vi "use photons for state.vi"(0 "state in":T1, 1 "apply measurement?":bool, 5 "location":T3, 7 "z-offset":i16, 9 "half valid z-range (ncycles * 64)":i16=500, 11 "scan radius":u16, 12 "tracking":bool) -> (4 "use photons to update tracker?":bool)   [LabVIEW 2010]
uses:
  kalman 3-axis state.ctl
  integrating single axis kalman state.ctl
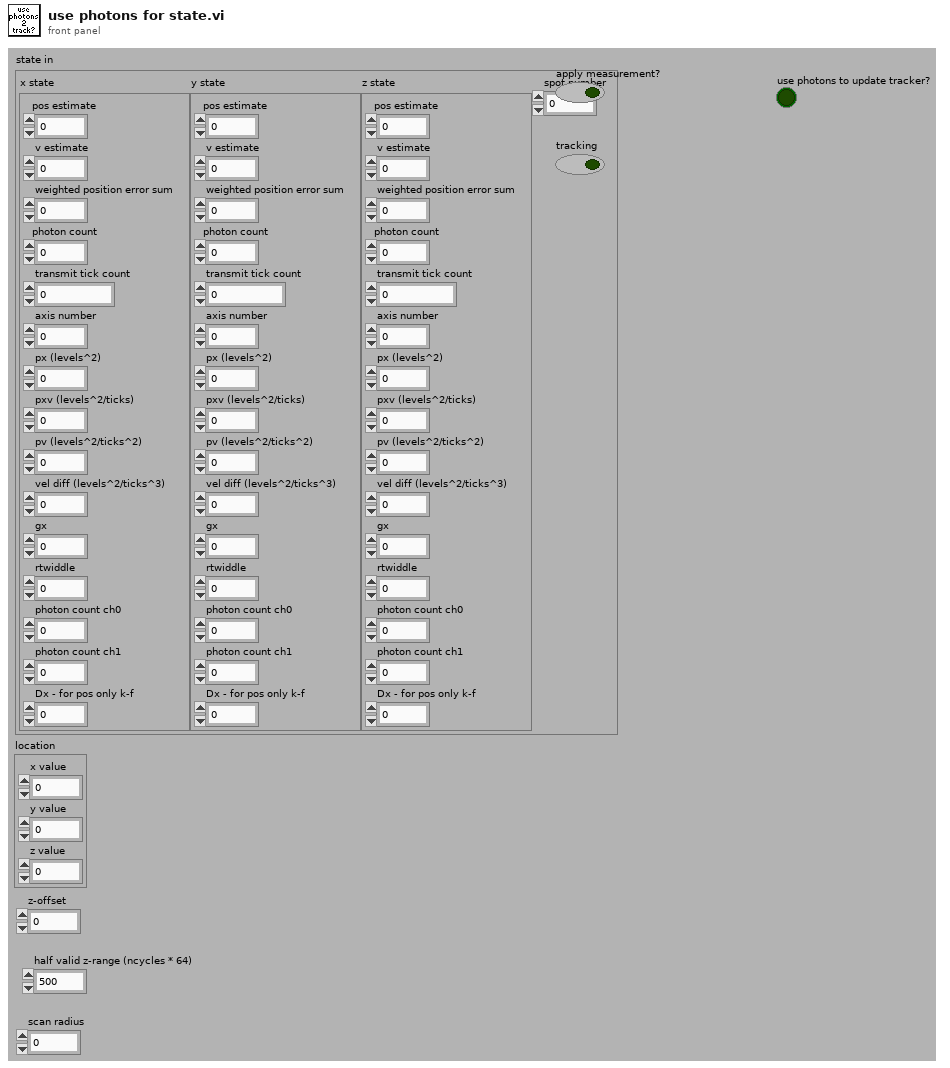
[diagram p1: front panel]
types:
  T1 = typedef "kalman 3-axis state.ctl" = cluster{"x state":T2, "y state":T2, "z state":T2, "spot number":u8}
  T2 = typedef "integrating single axis kalman state.ctl" = cluster{"pos estimate":fxp<+/-,32,16>, "v estimate":fxp<+/-,16,0>, "weighted position error sum":fxp<+/-,32,32>, "photon count":u32, "transmit tick count":u32, "axis number":u8, "px (levels^2)":fxp<+,32,19>, "pxv (levels^2/ticks)":fxp<+,32,2>, "pv (levels^2/ticks^2)":fxp<+,32,-14>, "vel diff (levels^2/ticks^3)":fxp<+,24,-22>, "gx":fxp<+,16,8>, "rtwiddle":fxp<+,16,26>, "photon count ch0":u32, "photon count ch1":u32, "Dx - for pos only k-f":fxp<+,32,19>}
  T3 = cluster{"x value":i16, "y value":i16, "z value":i16}
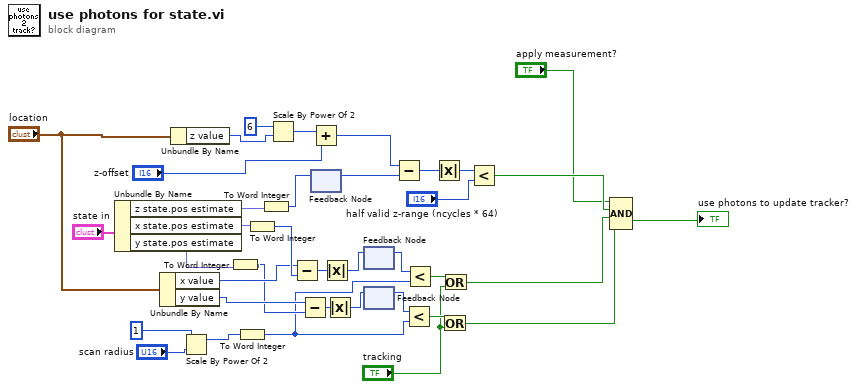
[diagram p0: block diagram]
diagram:
  n1 = Unbundle By Name("state in") -> ("z state.pos estimate"=w27:fxp<+/-,32,16>, "x state.pos estimate"=w25:fxp<+/-,32,16>, "y state.pos estimate"=w22:fxp<+/-,32,16>)
  n2 = Unbundle By Name("location") -> ("x value"=w23:i16, "y value"=w21:i16)
  n3 = Unbundle By Name("location") -> ("z value"=w30:i16)
  n4 = Scale By Power Of 2(n=1, x="scan radius") -> (x*2^n=w3:u16)
  n5 = To Word Integer(number=w22) -> (16bit integer=w20:i16)
  n6 = To Word Integer(number=w3) -> (16bit integer=w4:i16)
  n7 = To Word Integer(number=w25) -> (16bit integer=w24:i16)
  n8 = To Word Integer(number=w27) -> (16bit integer=w35:i16)
  n9 = Scale By Power Of 2(n=6, x=w30) -> (x*2^n=w29:i16)
  n10 = Subtract(x=w23, y=w24) -> (x-y=w19:i16)
  n11 = Subtract(x=w21, y=w20) -> (x-y=w18:i16)
  n12 = Add(x=w29, y="z-offset") -> (x+y=w28:i16)
  n13 = feedback-in #1(w35) -> ()
  n14 = feedback #1() -> (w8:i16)  [unwired: 1 in]
  n15 = Absolute Value(x=w19) -> (abs(x)=w10:i16)
  n16 = Absolute Value(x=w18) -> (abs(x)=w9:i16)
  n17 = feedback-in #2(w10) -> ()
  n18 = feedback #2() -> (w7:i16)  [unwired: 1 in]
  n19 = feedback-in #3(w9) -> ()
  n20 = feedback #3() -> (w6:i16)  [unwired: 1 in]
  n21 = Subtract(x=w28, y=w8) -> (x-y=w34:i16)
  n22 = Less?(x=w6, y=w4) -> (x < y?=w16:bool)
  n23 = Less?(x=w7, y=w4) -> (x < y?=w17:bool)
  n24 = Absolute Value(x=w34) -> (abs(x)=w33:i16)
  n25 = Or(x=w16, y="tracking") -> (x .or. y?=w12:bool)
  n26 = Or(x=w17, y="tracking") -> (x .or. y?=w13:bool)
  n27 = Less?(x=w33, y="half valid z-range (ncycles * 64)") -> (x < y?=w14:bool)
  n28 = Compound Arithmetic op=AND("apply measurement?", w14, w13, w12) -> (→"use photons to update tracker?":bool)
